vi "CélulaDessalinizadora2.0.vi"() -> ()   [LabVIEW 2014]
panel:
  out "String":string
  out "Tempo":dbl
  in  "Condutividade Máxima":dbl
  in  "NÚMERO DE CICLOS":dbl
  in  "Liga/Desliga":bool
  in  "Escolha: Porta Serial":refnum<visa-resource-name>="COM3"
  out "Dessorção":bool
  out "Adsorção":bool
  out "Single-Pass":bool
  out "Batch":bool
  in  "BATCH / SINGLE PASS":bool
  out "Potencial de Corte [V]":dbl(graph)
  out "pH":dbl(graph)
  out "Condutividade [us/cm]":dbl(graph)
  in  "?":T1(tab)
  in  "TEMPO DE ADSOR敲O P":dbl
  in  "CONDUTIVIDADE \nMÍNIMA NA ADSORÇÃO P":dbl
  in  "TEMPO DE DESSOR敲O P":dbl
  in  "CONDUTIVIDADE \nMÁXIMA NA DESSORÇÃO P":dbl
  in  "Selecionar parâmetro G":enum32{"Tempo", "Condutividade", "Potencial"}(tab)
  in  "TEMPO DE ADSOR敲O G":dbl
  in  "TEMPO DE DESSOR敲O G":dbl
  in  "CONDUTIVIDADE \nMÍNIMA NA ADSORÇÃO G":dbl
  in  "CONDUTIVIDADE \nMÁXIMA NA DESSORÇÃO G":dbl
  in  "POTENCIAL DE CORTE\nNA ADSOR敲O":dbl
  in  "POTENCIAL DE CORTE\nNA DESSOR敲O":dbl
  in  "POTENCIAL DE CORTE\nNA DESSOR敲O (V) G":dbl
  in  "CONDUTIVIDADE \nMÁXIMA NA DESSORÇÃO G 2":dbl
  in  "TEMPO DE DESSOR敲O G 2":dbl
  in  "TEMPO DE ADSOR敲O G 2":dbl
  in  "CONDUTIVIDADE \nMÍNIMA NA ADSORÇÃO G 2":dbl
  in  "POTENCIAL DE CORTE\nNA ADSOR敲O (V) G":dbl
  # "CONDUTIVIDADE MÁXIMA"
  # "s"
  # "us/cm"
  # "s"
  # "us/cm"
  # "s"
  # "s"
  # "us/cm"
  # "us/cm"
  # "VV"
  # "V"
  # "s"
  # "us/cm"
  # "VV"
  # "s"
  # "us/cm"
  # "VV"
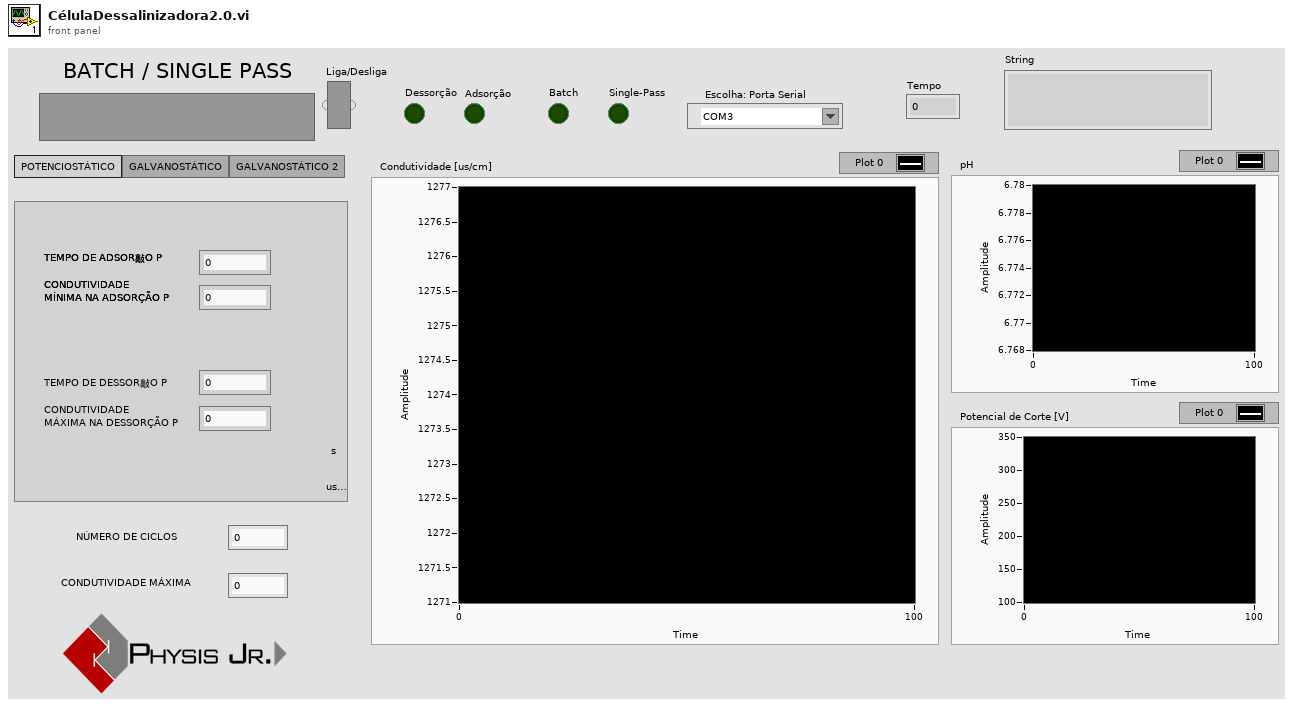
[diagram p1: front panel]
types:
  T1 = enum32{"POTENCIOSTÁTICO", "GALVANOSTÁTICO", "GALVANOSTÁTICO 2"}
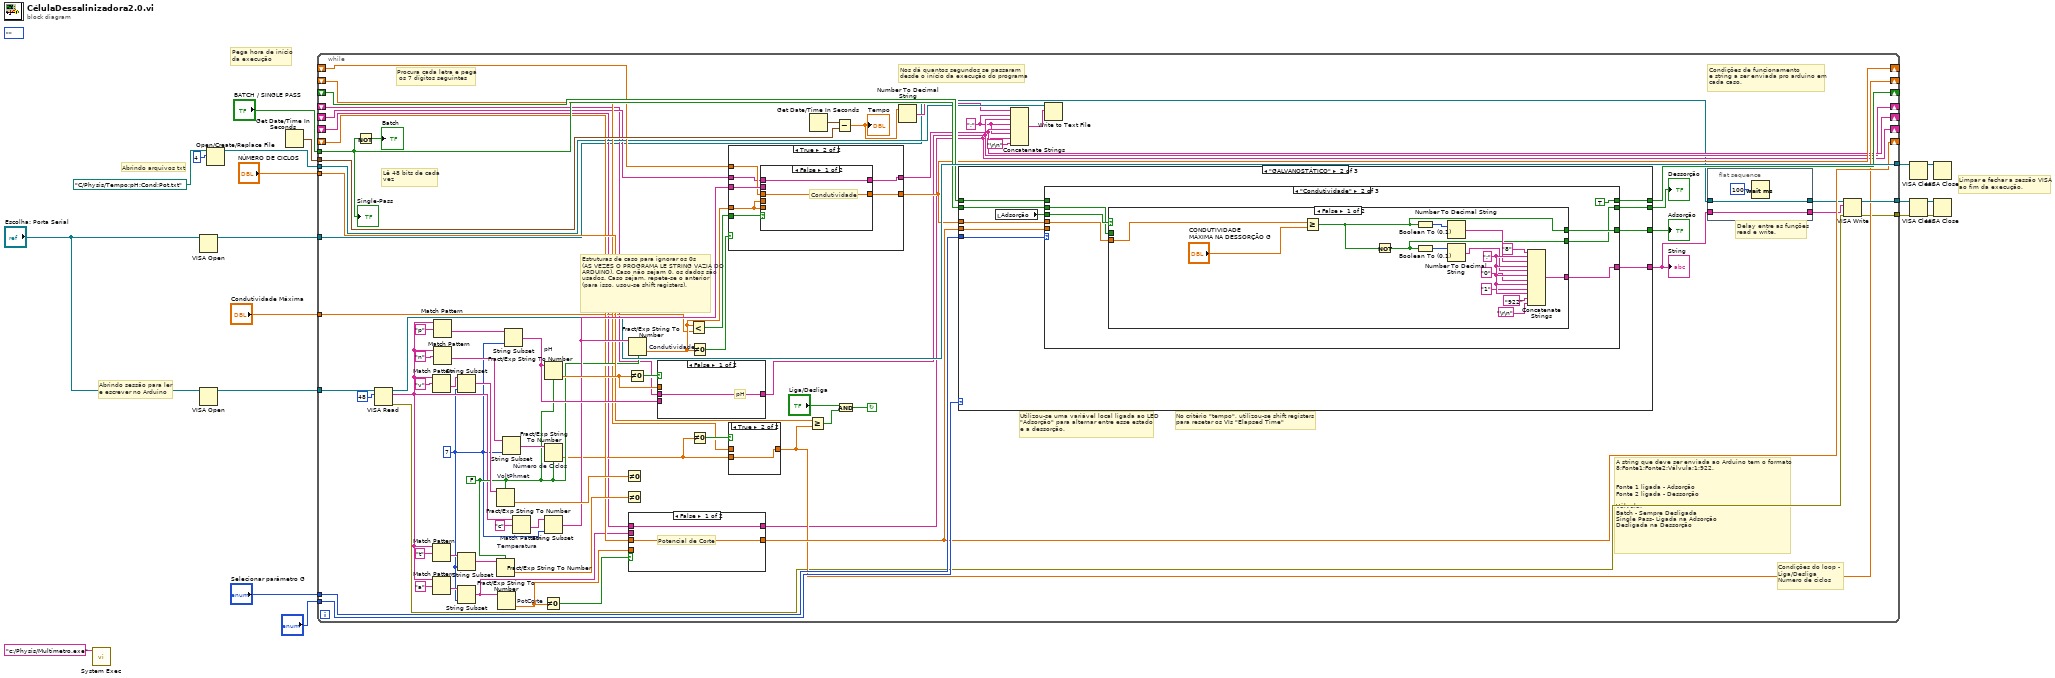
[diagram p0: block diagram]
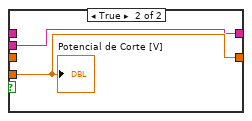
[diagram p3: hidden frame]
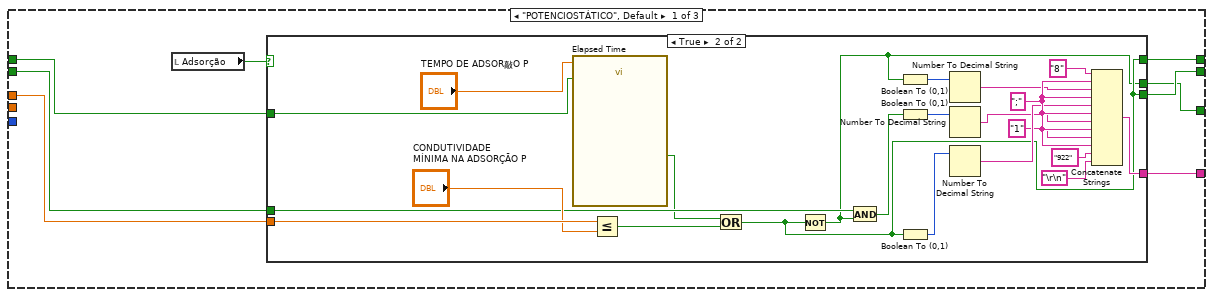
[diagram p4: hidden frame]
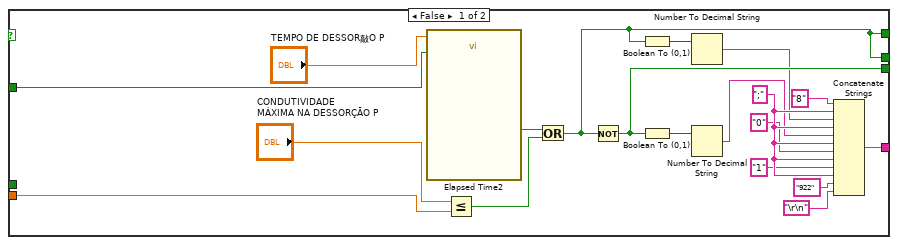
[diagram p5: hidden frame]
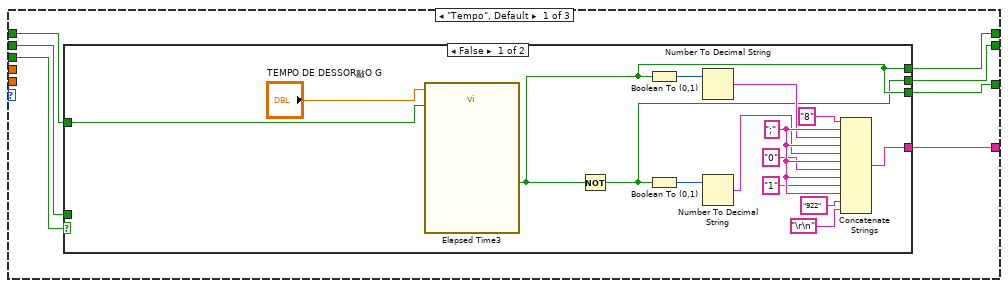
[diagram p6: hidden frame]
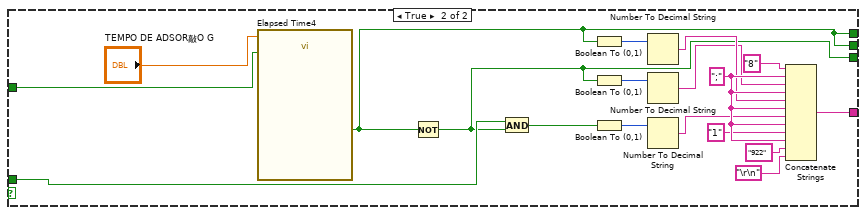
[diagram p7: hidden frame]
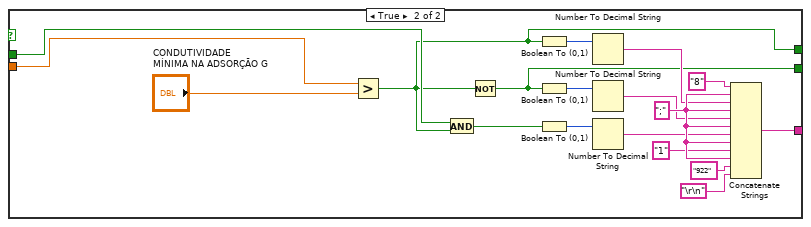
[diagram p8: hidden frame]
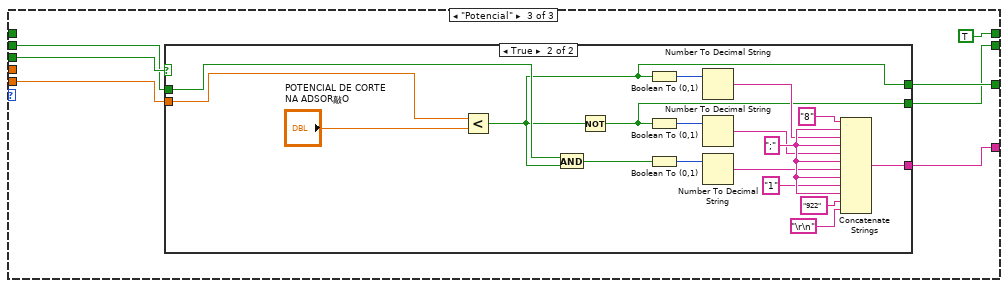
[diagram p9: hidden frame]
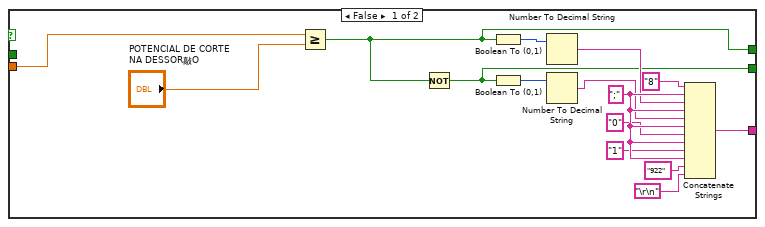
[diagram p10: hidden frame]
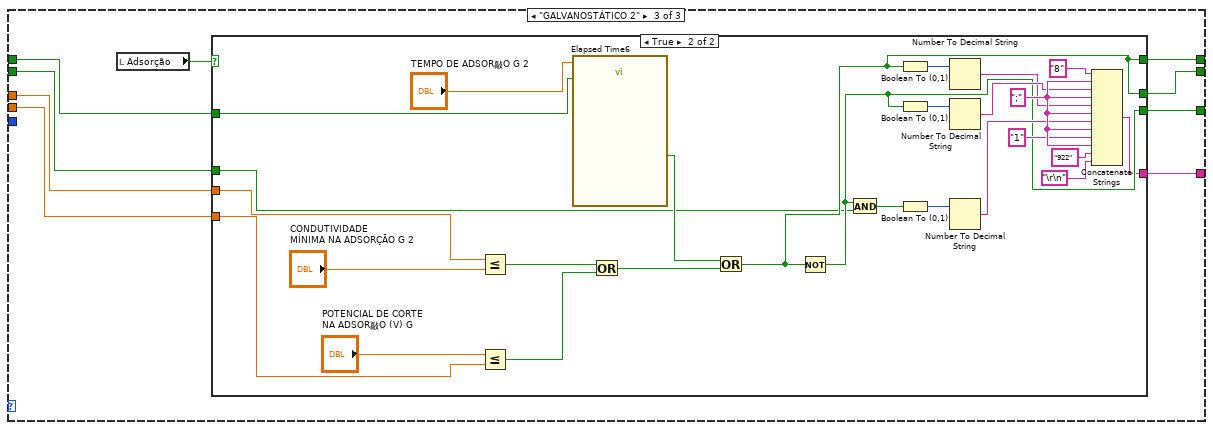
[diagram p11: hidden frame]
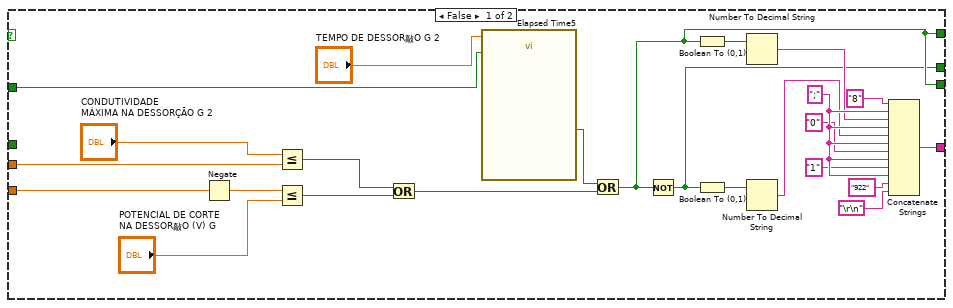
[diagram p12: hidden frame]
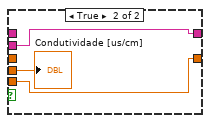
[diagram p14: hidden frame]
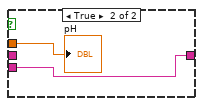
[diagram p15: hidden frame]
diagram:
  (unwired) enum16{""}.""
  # "Limpar e fechar a sessão VISA\nao fim da execução."
  # "Pega hora de início\nda execução"
  # "Abrindo arquivos txt"
  # "Abrindo sessão para ler \ne escrever no Arduino"
  n1 = call <vilib>:"System Exec.vi"("command line"="c:/Physis/Multímetro.exe") -> ()  [unwired: 7 in, 4 out]
  n2 = VISA Open(VISA resource name="Escolha: Porta Serial") -> (VISA resource name=w7:refnum<visa-resource-name>)  [unwired: 4 in, 1 out]
  n3 = VISA Open(VISA resource name="Escolha: Porta Serial") -> (VISA resource name=w17:refnum<visa-resource-name>)  [unwired: 4 in, 1 out]
  n4 = Open/Create/Replace File(file path (use dialog)=path "C:/Physis/Tempo;pH;Cond;Pot.txt", operation (0:open)=4) -> (refnum out=w15:refnum<file>)  [unwired: 4 in, 2 out]
  n5 = Get Date/Time In Seconds() -> (seconds since 1Jan1904=w16:timestamp)
  n6 = while {
    tunnel: w17 -> [w93]
    tunnel: w16 -> [w78]
    tunnel: w15 -> [w37]
    tunnel: "NÚMERO DE CICLOS" -> [w70]
    tunnel: [w69] -> w12
    tunnel: "?" -> [w65]
    tunnel: "Selecionar parâmetro G" -> [w64]
    tunnel: "BATCH / SINGLE PASS" -> [w62]
    shift-right: [w59] -> _
    shift-left: _ -> [w58]
    tunnel: w7 -> [w24]
    tunnel: [w57] -> w5
    shift-right: [w54] -> _
    shift-left: _ -> [w53]
    shift-right: [w52] -> _
    shift-left: _ -> [w51]
    shift-right: [w45] -> _
    shift-left: _ -> [w44]
    tunnel: "Condutividade Máxima" -> [w39]
    shift-right: [w35] -> _
    shift-left: _ -> [w34]
    shift-right: [w32] -> _
    shift-left: _ -> [w31]
    shift-right: [w29] -> _
    shift-left: _ -> [w28]
    tunnel: [w22] -> w2
    stop <- w43 continue-if-true
    w30 = ";"
    w68 = FALSE
    w49 = 7
    # "Delay entre as funções\nread e write."
    # "A string que deve ser enviada ao Arduino tem o formato \n8;Fonte1;Fonte2;Válvula;1;922.\n\n\nFonte 1 ligada - Adsorção\nFonte 2 ligada - Dessorção\n\nVálvula:\nBatch - Sempre Desligada\nSingle Pass- Ligada na Adsorção\nDesligada na Dessorção"
    # "Utilizou-se uma variável local ligada ao LED\n\"Adsorção\" para alternar entre esse estado\ne a dessorção."
    # "No critério \"tempo\", utilizou-se shift registers\npara resetar os VIs \"Elapsed Time\""
    # "Condições de funcionamento\ne string a ser enviada pro arduino em \ncada caso."
    # "Condições do loop - \nLiga/Desliga\nNúmero de ciclos"
    # "Estruturas de caso para ignorar os 0s\n(AS VEZES O PROGRAMA LE STRING VAZIA DO ARDUINO). Caso não sejam 0, os dados são usados. Caso sejam, repete-se o anterior (para isso, usou-se shift registers)."
    # "Procura cada letra e pega\n os 7 dígitos seguintes"
    # "Lê 48 bits de cada\nvez"
    # "Nos dá quantos segundos se passaram\ndesde o início da execução do programa"
    n7 = Not(x=w62) -> (.not. x?=→"Batch":bool)
    n8 = VISA Read(VISA resource name=w93, byte count=48) -> (VISA resource name out=w69:refnum<visa-resource-name>, read buffer=w67:string, error out=w23:errorcluster)  [unwired: 1 in, 1 out]
    n9 = Match Pattern(string=w67, regular expression="t") -> (after substring=w86:string)  [unwired: 1 in, 3 out]
    n10 = Match Pattern(string=w67, regular expression="v") -> (after substring=w83:string)  [unwired: 1 in, 3 out]
    n11 = Match Pattern(string=w67, regular expression="a") -> (after substring=w50:string)  [unwired: 1 in, 3 out]
    n12 = Match Pattern(string=w67, regular expression="p") -> (after substring=w87:string)  [unwired: 1 in, 3 out]
    n13 = Match Pattern(string=w67, regular expression="n") -> (after substring=w85:string)  [unwired: 1 in, 3 out]
    n14 = String Subset(string=w83, length (rest)=w49) -> (substring=w80:string)  [unwired: 1 in]
    n15 = String Subset(string=w86, length (rest)=w49) -> (substring=w82:string)  [unwired: 1 in]
    n16 = String Subset(string=w50, length (rest)=w49) -> (substring=w48:string)  [unwired: 1 in]
    n17 = Fract/Exp String To Number "VoltPhmet"(use system decimal point (T)=w68, string=w80) -> (number=w76:dbl)  [unwired: 2 in, 1 out]
    n18 = Fract/Exp String To Number "Temperatura"(use system decimal point (T)=w68, string=w82) -> (number=w77:dbl)  [unwired: 2 in, 1 out]
    n19 = Fract/Exp String To Number "PotCorte"(string=w48) -> (number=w55:dbl)  [unwired: 3 in, 1 out]
    n20 = String Subset(string=w85, length (rest)=w49) -> (substring=w81:string)  [unwired: 1 in]
    n21 = String Subset(string=w87, length (rest)=w49) -> (substring=w73:string)  [unwired: 1 in]
    n22 = Match Pattern(string=w67, regular expression="c") -> (after substring=w84:string)  [unwired: 1 in, 3 out]
    n23 = Fract/Exp String To Number "pH"(use system decimal point (T)=w68, string=w73) -> (number=w74:dbl)  [unwired: 2 in, 1 out]
    n24 = Fract/Exp String To Number "Número de Ciclos"(use system decimal point (T)=w68, string=w81) -> (number=w46:dbl)  [unwired: 2 in, 1 out]
    n25 = String Subset(string=w84, length (rest)=w49) -> (substring=w71:string)  [unwired: 1 in]
    n26 = Not Equal To 0?(x=w55) -> (x != 0?=w56:bool)
    n27 = Not Equal To 0?(x=w76) -> ()  [unwired: 1 out]
    n28 = Not Equal To 0?(x=w77) -> ()  [unwired: 1 out]
    n29 = Not Equal To 0?(x=w74) -> (x != 0?=w75:bool)
    n30 = Fract/Exp String To Number "Condutividade"(use system decimal point (T)=w68, string=w71) -> (number=w40:dbl)  [unwired: 2 in, 1 out]
    n31 = case shown="False" w56 {
      tunnel: w55 -> [_ w103]
      tunnel: [w101 w103] -> w54
      tunnel: w53 -> [w101 _]
      tunnel: w48 -> [_ w102]
      tunnel: [w100 w102] -> w29
      tunnel: w28 -> [w100 _]
      frame False {
        # "Potencial de Corte"
      }
      frame True {
        "Potencial de Corte [V]" <- w103
      }
    }
    n32 = case shown="False" w75 {
      tunnel: w74 -> [_ w358]
      tunnel: w73 -> [_ w357]
      tunnel: [w356 w357] -> w32
      tunnel: w31 -> [w356 _]
      frame False {
        # "pH"
      }
      frame True {
        "pH" <- w358
      }
    }
    n33 = Less?(x=w40, y=w39) -> (x < y?=w38:bool)
    n34 = Not Equal To 0?(x=w40) -> (x != 0?=w72:bool)
    n35 = Not Equal To 0?(x=w46) -> (x != 0?=w47:bool)
    n36 = case shown="True" w72 {
      tunnel: w40 -> [_ w347]
      tunnel: w71 -> [_ w350]
      tunnel: [w343 w348] -> w52
      tunnel: w51 -> [w343 w346]
      tunnel: w38 -> [_ w349]
      tunnel: [w342 w345] -> w35
      tunnel: w34 -> [w342 w344]
      frame False {
        # "Condutividade"
      }
      frame True {
        n37 = case shown="False" w349 {
          tunnel: w350 -> [_ w353]
          tunnel: w347 -> [_ w355]
          tunnel: [w352 w354] -> w348
          tunnel: w347 -> [_ w354]
          tunnel: w346 -> [w352 _]
          tunnel: [w351 w353] -> w345
          tunnel: w344 -> [w351 _]
          frame False {
            # "Condutividade"
          }
          frame True {
            "Condutividade [us/cm]" <- w355
          }
        }
      }
    }
    n38 = case shown="True" w47 {
      tunnel: [w98 w99] -> w45
      tunnel: w46 -> [_ w99]
      tunnel: w44 -> [w98 _]
      frame False {
      }
      frame True {
      }
    }
    n39 = Greater Or Equal?(x=w70, y=w45) -> (x >= y?=w41:bool)
    n40 = Get Date/Time In Seconds() -> (seconds since 1Jan1904=w79:timestamp)
    n41 = Subtract(x=w79, y=w78) -> (x-y=w21:dbl)
    "Tempo" <- w21
    n42 = And(x="Liga/Desliga", y=w41) -> (x .and. y?=w43:bool)
    n43 = Number To Decimal String(number=w21) -> (decimal integer string=w36:string)  [unwired: 1 in]
    n44 = case shown="\"GALVANOSTÁTICO\"" w65 {
      tunnel: w54 -> [_ w162 w288]
      tunnel: w52 -> [w109 w161 w289]
      tunnel: w58 -> [w108 w160 w290]
      tunnel: [w110 w159 w285] -> w59
      tunnel: [w104 w158 w286] -> w61
      tunnel: [w105 w157 w287] -> w60
      tunnel: [w107 w156 w283] -> w20
      tunnel: w62 -> [w106 w155 w284]
      tunnel: w64 -> [_ w154 _]
      frame "POTENCIOSTÁTICO", Default {
        n45 = local read "Adsorção"() -> (w111:bool)
        n46 = case shown="True" w111 {
          tunnel: [w115 w135] -> w110
          tunnel: w109 -> [w127 w152]
          tunnel: w108 -> [w130 w148]
          tunnel: [w116 w139] -> w107
          tunnel: w106 -> [_ w138]
          tunnel: [w118 w135] -> w105
          tunnel: [w115 w134] -> w104
          frame False {
            w122 = ";"
            n47 = call "Elapsed Time2"("Time Target (s)"="TEMPO DE DESSOR敲O P", "Reset"=w130) -> ("Time has Elapsed"=w126:bool)  [unwired: 10 in, 7 out]
            n48 = Less Or Equal?(x="CONDUTIVIDADE \nMÁXIMA NA DESSORÇÃO P", y=w127) -> (x <= y?=w125:bool)
            n49 = Or(x=w126, y=w125) -> (x .or. y?=w115:bool)
            n50 = Not(x=w115) -> (.not. x?=w118:bool)
            n51 = Boolean To (0,1)(Boolean=w115) -> (0, 1=w120:i16)
            n52 = Boolean To (0,1)(Boolean=w118) -> (0, 1=w121:i16)
            n53 = Number To Decimal String(number=w120) -> (decimal integer string=w114:string)  [unwired: 1 in]
            n54 = Number To Decimal String(number=w121) -> (decimal integer string=w113:string)  [unwired: 1 in]
            n55 = Concatenate Strings("8", w122, w114, w122, w113, w122, "0", w122, "1", w122, "922", "\r\n") -> (w116:string)
          }
          frame True {
            w144 = ";"
            n56 = call "Elapsed Time"("Time Target (s)"="TEMPO DE ADSOR敲O P", "Reset"=w148) -> ("Time has Elapsed"=w136:bool)  [unwired: 10 in, 7 out]
            n57 = Less Or Equal?(x=w152, y="CONDUTIVIDADE \nMÍNIMA NA ADSORÇÃO P") -> (x <= y?=w150:bool)
            n58 = Or(x=w136, y=w150) -> (x .or. y?=w135:bool)
            n59 = Not(x=w135) -> (.not. x?=w134:bool)
            n60 = And(x=w138, y=w134) -> (x .and. y?=w137:bool)
            n61 = Boolean To (0,1)(Boolean=w134) -> (0, 1=w132:i16)
            n62 = Boolean To (0,1)(Boolean=w137) -> (0, 1=w147:i16)
            n63 = Boolean To (0,1)(Boolean=w135) -> (0, 1=w133:i16)
            n64 = Number To Decimal String(number=w132) -> (decimal integer string=w142:string)  [unwired: 1 in]
            n65 = Number To Decimal String(number=w147) -> (decimal integer string=w141:string)  [unwired: 1 in]
            n66 = Number To Decimal String(number=w133) -> (decimal integer string=w143:string)  [unwired: 1 in]
            n67 = Concatenate Strings("8", w144, w142, w144, w143, w144, w141, w144, "1", w144, "922", "\r\n") -> (w139:string)
          }
        }
      }
      frame "GALVANOSTÁTICO" {
        n68 = local read "Adsorção"() -> (w153:bool)
        n69 = case shown="\"Condutividade\"" w154 {
          tunnel: w153 -> [w169 w209 w249]
          tunnel: w162 -> [_ _ w248]
          tunnel: w161 -> [_ w208 _]
          tunnel: w160 -> [w168 _ _]
          tunnel: [w167 TRUE TRUE] -> w159
          tunnel: [w166 w205 w245] -> w158
          tunnel: [w165 w204 w244] -> w157
          tunnel: [w164 w207 w246] -> w156
          tunnel: w155 -> [w163 w206 w247]
          frame "Tempo", Default {
            n70 = case shown="False" w169 {
              tunnel: w168 -> [w184 w202]
              tunnel: [w175 w188] -> w167
              tunnel: [w175 w191] -> w166
              tunnel: [w174 w188] -> w165
              tunnel: [w172 w189] -> w164
              tunnel: w163 -> [_ w192]
              frame False {
                w181 = ";"
                n71 = call "Elapsed Time3"("Time Target (s)"="TEMPO DE DESSOR敲O G", "Reset"=w184) -> ("Time has Elapsed"=w175:bool)  [unwired: 10 in, 7 out]
                n72 = Not(x=w175) -> (.not. x?=w174:bool)
                n73 = Boolean To (0,1)(Boolean=w175) -> (0, 1=w180:i16)
                n74 = Boolean To (0,1)(Boolean=w174) -> (0, 1=w179:i16)
                n75 = Number To Decimal String(number=w180) -> (decimal integer string=w177:string)  [unwired: 1 in]
                n76 = Number To Decimal String(number=w179) -> (decimal integer string=w178:string)  [unwired: 1 in]
                n77 = Concatenate Strings("8", w181, w177, w181, w178, w181, "0", w181, "1", w181, "922", "\r\n") -> (w172:string)
              }
              frame True {
                w198 = ";"
                n78 = call "Elapsed Time4"("Time Target (s)"="TEMPO DE ADSOR敲O G", "Reset"=w202) -> ("Time has Elapsed"=w188:bool)  [unwired: 10 in, 7 out]
                n79 = Not(x=w188) -> (.not. x?=w191:bool)
                n80 = And(x=w192, y=w191) -> (x .and. y?=w190:bool)
                n81 = Boolean To (0,1)(Boolean=w188) -> (0, 1=w196:i16)
                n82 = Boolean To (0,1)(Boolean=w191) -> (0, 1=w197:i16)
                n83 = Boolean To (0,1)(Boolean=w190) -> (0, 1=w201:i16)
                n84 = Number To Decimal String(number=w196) -> (decimal integer string=w195:string)  [unwired: 1 in]
                n85 = Number To Decimal String(number=w197) -> (decimal integer string=w186:string)  [unwired: 1 in]
                n86 = Number To Decimal String(number=w201) -> (decimal integer string=w194:string)  [unwired: 1 in]
                n87 = Concatenate Strings("8", w198, w186, w198, w195, w198, w194, w198, "1", w198, "922", "\r\n") -> (w189:string)
              }
            }
          }
          frame "Condutividade" {
            n88 = case shown="False" w209 {
              tunnel: w208 -> [w224 w242]
              tunnel: [w214 w231] -> w207
              tunnel: w206 -> [_ w229]
              tunnel: [w213 w228] -> w205
              tunnel: [w212 w227] -> w204
              frame False {
                w221 = ";"
                n89 = Greater Or Equal?(x=w224, y="CONDUTIVIDADE \nMÁXIMA NA DESSORÇÃO G") -> (x >= y?=w213:bool)
                n90 = Not(x=w213) -> (.not. x?=w212:bool)
                n91 = Boolean To (0,1)(Boolean=w213) -> (0, 1=w220:i16)
                n92 = Boolean To (0,1)(Boolean=w212) -> (0, 1=w219:i16)
                n93 = Number To Decimal String(number=w220) -> (decimal integer string=w217:string)  [unwired: 1 in]
                n94 = Number To Decimal String(number=w219) -> (decimal integer string=w218:string)  [unwired: 1 in]
                n95 = Concatenate Strings("8", w221, w217, w221, w218, w221, "0", w221, "1", w221, "922", "\r\n") -> (w214:string)
              }
              frame True {
                w238 = ";"
                n96 = Greater?(x=w242, y="CONDUTIVIDADE \nMÍNIMA NA ADSORÇÃO G") -> (0:w228:bool)
                n97 = And(x=w229, y=w228) -> (x .and. y?=w230:bool)
                n98 = Not(x=w228) -> (.not. x?=w227:bool)
                n99 = Boolean To (0,1)(Boolean=w228) -> (0, 1=w237:i16)
                n100 = Boolean To (0,1)(Boolean=w227) -> (0, 1=w236:i16)
                n101 = Boolean To (0,1)(Boolean=w230) -> (0, 1=w241:i16)
                n102 = Number To Decimal String(number=w237) -> (decimal integer string=w234:string)  [unwired: 1 in]
                n103 = Number To Decimal String(number=w236) -> (decimal integer string=w235:string)  [unwired: 1 in]
                n104 = Number To Decimal String(number=w241) -> (decimal integer string=w233:string)  [unwired: 1 in]
                n105 = Concatenate Strings("8", w238, w234, w238, w235, w238, w233, w238, "1", w238, "922", "\r\n") -> (w231:string)
              }
            }
          }
          frame "Potencial" {
            n106 = case shown="True" w249 {
              tunnel: w248 -> [w264 w282]
              tunnel: w247 -> [_ w270]
              tunnel: [w254 w269] -> w246
              tunnel: [w253 w268] -> w245
              tunnel: [w252 w267] -> w244
              frame False {
                w261 = ";"
                n107 = Greater Or Equal?(x=w264, y="POTENCIAL DE CORTE\nNA DESSOR敲O") -> (x >= y?=w253:bool)
                n108 = Not(x=w253) -> (.not. x?=w252:bool)
                n109 = Boolean To (0,1)(Boolean=w253) -> (0, 1=w260:i16)
                n110 = Boolean To (0,1)(Boolean=w252) -> (0, 1=w259:i16)
                n111 = Number To Decimal String(number=w260) -> (decimal integer string=w257:string)  [unwired: 1 in]
                n112 = Number To Decimal String(number=w259) -> (decimal integer string=w258:string)  [unwired: 1 in]
                n113 = Concatenate Strings("8", w261, w257, w261, w258, w261, "0", w261, "1", w261, "922", "\r\n") -> (w254:string)
              }
              frame True {
                w278 = ";"
                n114 = Less?(x=w282, y="POTENCIAL DE CORTE\nNA ADSOR敲O") -> (x < y?=w268:bool)
                n115 = And(x=w270, y=w268) -> (x .and. y?=w271:bool)
                n116 = Not(x=w268) -> (.not. x?=w267:bool)
                n117 = Boolean To (0,1)(Boolean=w268) -> (0, 1=w277:i16)
                n118 = Boolean To (0,1)(Boolean=w267) -> (0, 1=w276:i16)
                n119 = Boolean To (0,1)(Boolean=w271) -> (0, 1=w281:i16)
                n120 = Number To Decimal String(number=w277) -> (decimal integer string=w274:string)  [unwired: 1 in]
                n121 = Number To Decimal String(number=w276) -> (decimal integer string=w275:string)  [unwired: 1 in]
                n122 = Number To Decimal String(number=w281) -> (decimal integer string=w273:string)  [unwired: 1 in]
                n123 = Concatenate Strings("8", w278, w274, w278, w275, w278, w273, w278, "1", w278, "922", "\r\n") -> (w269:string)
              }
            }
          }
        }
      }
      frame "GALVANOSTÁTICO 2" {
        n124 = local read "Adsorção"() -> (w291:bool)
        n125 = case shown="True" w291 {
          tunnel: w290 -> [w314 w340]
          tunnel: w289 -> [w311 w339]
          tunnel: w288 -> [w313 w336]
          tunnel: [w293 w323] -> w287
          tunnel: [w294 w319] -> w286
          tunnel: [w294 w323] -> w285
          tunnel: w284 -> [_ w318]
          tunnel: [w295 w317] -> w283
          frame False {
            w302 = ";"
            n126 = Negate(x=w313) -> (-x=w306:dbl)
            n127 = Less Or Equal?(x="CONDUTIVIDADE \nMÁXIMA NA DESSORÇÃO G 2", y=w311) -> (x <= y?=w310:bool)
            n128 = Less Or Equal?(x=w306, y="POTENCIAL DE CORTE\nNA DESSOR敲O (V) G") -> (x <= y?=w309:bool)
            n129 = Or(x=w310, y=w309) -> (x .or. y?=w307:bool)
            n130 = call "Elapsed Time5"("Time Target (s)"="TEMPO DE DESSOR敲O G 2", "Reset"=w314) -> ("Time has Elapsed"=w308:bool)  [unwired: 10 in, 7 out]
            n131 = Or(x=w308, y=w307) -> (x .or. y?=w294:bool)
            n132 = Not(x=w294) -> (.not. x?=w293:bool)
            n133 = Boolean To (0,1)(Boolean=w294) -> (0, 1=w301:i16)
            n134 = Boolean To (0,1)(Boolean=w293) -> (0, 1=w300:i16)
            n135 = Number To Decimal String(number=w301) -> (decimal integer string=w299:string)  [unwired: 1 in]
            n136 = Number To Decimal String(number=w300) -> (decimal integer string=w297:string)  [unwired: 1 in]
            n137 = Concatenate Strings("8", w302, w299, w302, w297, w302, "0", w302, "1", w302, "922", "\r\n") -> (w295:string)
          }
          frame True {
            w329 = ";"
            n138 = Less Or Equal?(x=w339, y="CONDUTIVIDADE \nMÍNIMA NA ADSORÇÃO G 2") -> (x <= y?=w335:bool)
            n139 = Less Or Equal?(x="POTENCIAL DE CORTE\nNA ADSOR敲O (V) G", y=w336) -> (x <= y?=w334:bool)
            n140 = call "Elapsed Time6"("Time Target (s)"="TEMPO DE ADSOR敲O G 2", "Reset"=w340) -> ("Time has Elapsed"=w333:bool)  [unwired: 10 in, 7 out]
            n141 = Or(x=w335, y=w334) -> (x .or. y?=w332:bool)
            n142 = Or(x=w333, y=w332) -> (x .or. y?=w323:bool)
            n143 = Not(x=w323) -> (.not. x?=w319:bool)
            n144 = And(x=w319, y=w318) -> (x .and. y?=w321:bool)
            n145 = Boolean To (0,1)(Boolean=w323) -> (0, 1=w327:i16)
            n146 = Boolean To (0,1)(Boolean=w319) -> (0, 1=w328:i16)
            n147 = Boolean To (0,1)(Boolean=w321) -> (0, 1=w322:i16)
            n148 = Number To Decimal String(number=w327) -> (decimal integer string=w324:string)  [unwired: 1 in]
            n149 = Number To Decimal String(number=w328) -> (decimal integer string=w326:string)  [unwired: 1 in]
            n150 = Number To Decimal String(number=w322) -> (decimal integer string=w320:string)  [unwired: 1 in]
            n151 = Concatenate Strings("8", w329, w326, w329, w324, w329, w320, w329, "1", w329, "922", "\r\n") -> (w317:string)
          }
        }
      }
    }
    "Adsorção" <- w61
    "Dessorção" <- w60
    "String" <- w20
    n152 = Concatenate Strings(w36, w30, w32, w30, w35, w30, w29, "\r\n") -> (w27:string)
    n153 = Write to Text File(file (use dialog)=w37, text=w27) -> ()  [unwired: 2 in, 3 out]
    n154 = flat-sequence {
      tunnel: w20 -> [w97]
      tunnel: [w97] -> w26
      tunnel: [w96] -> w25
      tunnel: w24 -> [w96]
      frame #0 {
        n155 = Wait (ms)(milliseconds to wait=100) -> ()  [unwired: 1 out]
      }
    }
    n156 = VISA Write(VISA resource name=w25, write buffer=w26, error in (no error)=w23) -> (VISA resource name out=w57:refnum<visa-resource-name>, error out=w22:errorcluster)  [unwired: 1 out]
    "Single-Pass" <- w62
  }
  n157 = VISA Clear(VISA resource name=w12) -> (VISA resource name out=w13:refnum<visa-resource-name>)  [unwired: 1 in, 1 out]
  n158 = VISA Clear(VISA resource name=w5, error in (no error)=w2) -> (VISA resource name out=w6:refnum<visa-resource-name>, error out=w1:errorcluster)
  n159 = VISA Close(VISA resource name=w13) -> ()  [unwired: 1 in, 1 out]
  n160 = VISA Close(VISA resource name=w6, error in (no error)=w1) -> ()  [unwired: 1 out]
